vi "CalcBusLoad.vi"(8 "error in":errorcluster, 11 "UpdateDelay [ms]":u32) -> (0 "error out":errorcluster, 2 "BusLoad":dbl, 3 "Peak Bus Load":dbl)   [LabVIEW 2014, in "CAN Bus Monitor Engine.lvlib"]
uses:
  CAN Bus Monitor Engine.lvlib
  Controls/Set Dyn Vars.ctl
  BM Global Vars.vi
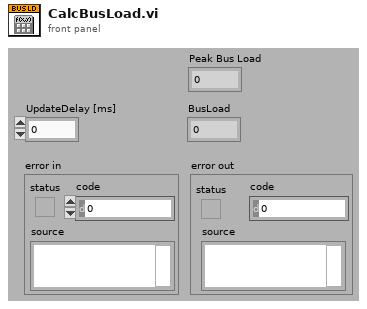
[diagram p1: front panel]
types:
  T1 = cluster{"IncMinFrameTime":dbl, "IncMaxFrameTime":dbl, "Min Frame Length":dbl[][], "Max Frame Length":dbl[][], "Std Frames":u32, "Ext Frames":u32, "Error Frames":u32, "Remote Frames":u32, "Std Frames / Sec":u32, "Ext Frames / Sec":u32, "Error Frames / Sec":u32, "Remote Frames / Sec":u32, "Peak Bus Load":dbl, "Bus Load":dbl, "Start Timestamp":dbl, "Null Frames":u32, "Null Frames / Sec":u32}
  T2 = typedef "CAN Bus Monitor Engine.lvlib/Set Dyn Vars.ctl" = enum16{"Std Frames", "Std Frames / Sec", "Ext Frames", "Ext Frames / Sec", "Remote Frames", "Remote Frames / Sec", "Error Frames", "Error Frames / Sec", "BusLoad", "SumFrames", "SumFrames / Sec", "Null Frames", "Null Frames / Sec", "Peak Bus Load", "State", "IncMinFrameTime", "IncMaxFrameTime", "Driver Status", "CAN Comm State", "LIN Comm State", "FlexRay Comm State"}
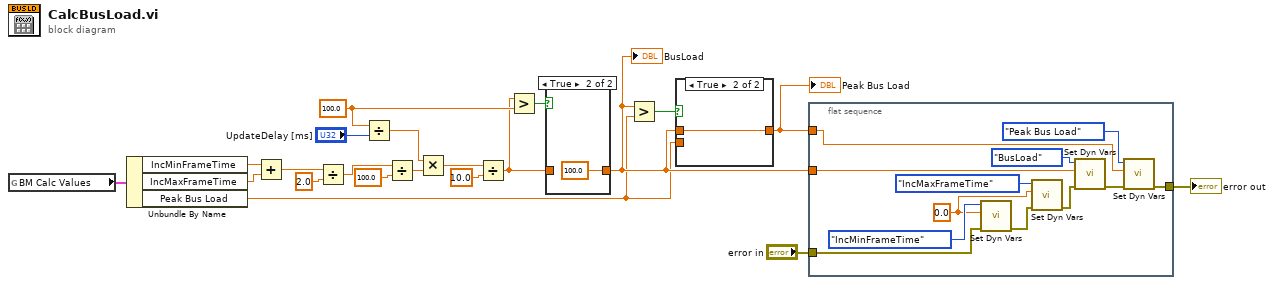
[diagram p0: block diagram]
diagram:
  w10 = 100.0
  n1 = global read "BM Global Vars.vi" "BM Calc Values"() -> (w5:T1)
  n2 = Unbundle By Name(w5) -> ("IncMinFrameTime"=w18:dbl, "IncMaxFrameTime"=w17:dbl, "Peak Bus Load"=w3:dbl)
  n3 = Add(x=w18, y=w17) -> (x+y=w16:dbl)
  n4 = Divide(x=w16, y=2.0) -> (x/y=w14:dbl)
  n5 = Divide(x=w10, y="UpdateDelay [ms]") -> (x/y=w12:dbl)
  n6 = Divide(x=w14, y=100.0) -> (x/y=w11:dbl)
  n7 = Multiply(x=w12, y=w11) -> (x*y=w7:dbl)
  n8 = Divide(x=w7, y=10.0) -> (x/y=w6:dbl)
  n9 = Greater?(x=w6, y=w10) -> (0:w9:bool)
  n10 = case shown="True" w9 {
    tunnel: [w22 100.0] -> w20
    tunnel: w6 -> [w22 _]
    frame False {
    }
    frame True {
    }
  }
  "BusLoad" <- w20
  n11 = Greater?(x=w20, y=w3) -> (0:w4:bool)
  n12 = case shown="True" w4 {
    tunnel: [w24 w25] -> w1
    tunnel: w20 -> [_ w25]
    tunnel: w3 -> [w24 _]
    frame False {
    }
    frame True {
    }
  }
  "Peak Bus Load" <- w1
  n13 = flat-sequence {
    tunnel: w20 -> [w33]
    tunnel: w1 -> [w31]
    tunnel: [w26] -> w19
    tunnel: "error in" -> [w27]
    frame #0 {
      w36 = 0.0 ("IncMinFrameTime")
      n14 = call "Set Dyn Vars.vi"("error in"=w27, "Data"=w36, "Set Values"=Set_Dyn_Vars."IncMinFrameTime") -> ("error out"=w30:errorcluster)  [unwired: 8 in]
      n15 = call "Set Dyn Vars.vi"("error in"=w30, "Data"=w36, "Set Values"=Set_Dyn_Vars."IncMaxFrameTime") -> ("error out"=w29:errorcluster)  [unwired: 8 in]
      n16 = call "Set Dyn Vars.vi"("error in"=w29, "Data"=w33, "Set Values"=Set_Dyn_Vars."BusLoad") -> ("error out"=w28:errorcluster)  [unwired: 8 in]
      n17 = call "Set Dyn Vars.vi"("error in"=w28, "Data"=w31, "Set Values"=Set_Dyn_Vars."Peak Bus Load") -> ("error out"=w26:errorcluster)  [unwired: 8 in]
    }
  }
  "error out" <- w19
